vi "Math-Update Average.vi"(3 "Navg In":i32, 4 "New sample":dbl[](array[numeric]), 5 "Avg In":dbl[](array[numeric])) -> (0 "Navg Out":i32, 2 "Avg Out":dbl[](array[numeric]))   [LabVIEW 2015]
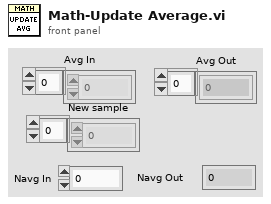
[diagram p1: front panel]
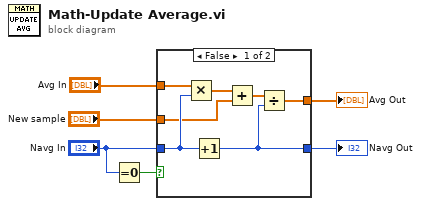
[diagram p0: block diagram]
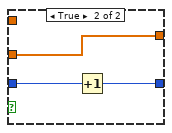
[diagram p2: hidden frame]
diagram:
  n1 = Equal To 0?(x="Navg In") -> (x = 0?=w5:bool)
  n2 = case shown="False" w5 {
    tunnel: "Avg In" -> [w13 _]
    tunnel: [w7 w14] -> w4
    tunnel: "Navg In" -> [w12 w16]
    tunnel: [w8 w15] -> w2
    tunnel: "New sample" -> [w10 w14]
    frame False {
      n3 = Multiply(x=w13, y=w12) -> (x*y=w11:dbl[])
      n4 = Increment(x=w12) -> (x+1=w8:i32)
      n5 = Add(x=w11, y=w10) -> (x+y=w9:dbl[])
      n6 = Divide(x=w9, y=w8) -> (x/y=w7:dbl[])
    }
    frame True {
      n7 = Increment(x=w16) -> (x+1=w15:i32)
    }
  }
  "Avg Out" <- w4
  "Navg Out" <- w2
